vi "Drive_Begin.vi"   [LabVIEW 2019]
uses:
  Drive_Cluster.ctl
  Drive_States.ctl
  Drive_Globals.vi
types:
  T1 = typedef "Drive_Cluster.ctl" = cluster{"Control_State":T2, "Angular_Throttle":dbl, "Linear_Throttle":dbl, "Torque_Changing":bool, "Step":dbl, "Parameter_1":dbl, "Parameter_2":dbl, "Parameter_3":dbl, "Parameter_4":dbl, "Auto_Notifier":refnum<notifier>}
  T2 = typedef "Drive_States.ctl" = enum16{"Percent_Voltage_Control", "Speed_Control", "Curvature_Control", "Command_HeadingDistance", "Command_TurnToHeading", "Command_FollowPath"}
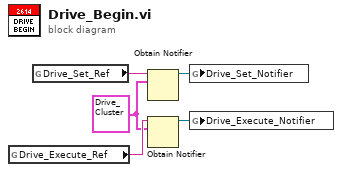
[diagram p0: block diagram]
diagram:
  w3 = T1 {"Control_State"=enum."Percent_Voltage_Control", "Angular_Throttle"=0.0, "Linear_Throttle"=0.0, "Torque_Changing"=FALSE, "Step"=0.0, "Parameter_1"=0.0, "Parameter_2"=0.0, "Parameter_3"=0.0, "Parameter_4"=0.0, "Auto_Notifier"=refnum} ("Drive_Cluster")
  n1 = global read "Drive_Globals.vi" "Drive_Execute_Ref"() -> (w5:string)
  n2 = global read "Drive_Globals.vi" "Drive_Set_Ref"() -> (w4:string)
  n3 = Obtain Notifier(name (unnamed)=w4, notification data type=w3) -> (notifier out=w1:refnum<notifier>)  [unwired: 2 in, 2 out]
  n4 = Obtain Notifier(name (unnamed)=w5, notification data type=w3) -> (notifier out=w2:refnum<notifier>)  [unwired: 2 in, 2 out]
  n5 = global write "Drive_Globals.vi" "Drive_Set_Notifier"(w1) -> ()
  n6 = global write "Drive_Globals.vi" "Drive_Execute_Notifier"(w2) -> ()
